vi "OCT with WavePond Clock periodic save updated.vi"() -> ()   [LabVIEW 2014]
doc: "I. Description:\nThis example demonstrates how to acquire a continuous amount of data (Waveform) using the DAQ device's internal clock.\n\nII. Instructions for Running:\n1. Create an analog input voltage channel.\n2. Set the rate for the sample clock. Additionally, define the sample mode to be continuous.\n3. Call the Start VI to start the acquisition.\n4. Read the waveform data in a loop until the user hits the stop button or an error occurs.\nNote: This example reads data from one or more channels and returns an array of data. Use the Index Array function to access an individual channel of data.\n5. Call the Clear Task VI to clear the Task.\n6. Use the popup dialog box to display an error if any.\n\nIV. I/O Connections Overview:\nMake sure your signal input terminal matches the Physical Channel I/O Control. For further connection information, refer to your hardware reference manual."
uses:
  ATS-VI/ATS_ctl/Device_Ctrl.ctl
  ATS-VI/ATS_ctl/ATS_Async_Ctrl.ctl
  ATS-VI/ATS_ctl/ATS_Async_Mode.ctl
  ATS-VI/ATS_ctl/ATS_DMA_Channel.ctl
  ATS-VI/ATS_ctl/ATS_ReadSamples.ctl
  ATS-VI/ATS_ctl/ATS_Check_Ctrl.ctl
  ATS-VI/ATS_ctl/ClockSource.ctl
  Galvo VIs/galvo_states.ctl
  Signal Processing/processing_states.ctl
  En Face/En Face States.ctl
  Saving Data/Saving Data States.ctl
  Type Defs/OCT Hardware States.ctl
  ATS-VI/ATS_ctl/Range.ctl
  ATS-VI/ATS_ctl/Impedance.ctl
  Type Defs/OCT Imaging Parameters Cluster.ctl
  Signal Processing/Display Raw Data states.ctl
  ATS-VI/ATS_ctl/ATS_Spec_Selector.ctl
  Classes/Galvo/Scanning Cluster.ctl
  Classes/Galvo/Galvo.lvclass
  Type Defs/OCT DAQ Channel Data Type.ctl
  Type Defs/Display States.ctl
  ATS-VI/ATS_ctl/Coupling.ctl
  ATS-VI/ATS_ctl/Bandwidth.ctl
  ATS-VI/ATS_ctl/InputCtrl.ctl
  ATS-VI/ATS_ctl/TriggerEngine.ctl
  ATS-VI/ATS_ctl/ExtTrigRange.ctl
  ATS-VI/ATS_ctl/ExtTrigger.ctl
  ATS-VI/ATS_ctl/TriggerOperation.ctl
  ATS-VI/ATS_ctl/Trigger.ctl
  ATS-VI/ATS_ctl/ClockRate.ctl
  ATS-VI/ATS_ctl/ClockEdge.ctl
  ATS-VI/ATS_ctl/Clock.ctl
  ATS-VI/ATS_ctl/Record.ctl
  ATS-VI/ATS_ctl/ATS_Global.ctl
  ATS-VI/ATS_ctl/ATS_Async_Status.ctl
  En Face/En Face Depth Parameters.ctl
  ATS-VI/ATS_ctl/ATS_Async_Setting.ctl
panel:
  in  "update en face image?":bool=TRUE
  in  "total measurement time":dbl=28800.0
  in  "save every ? second":dbl=60.0
  out "First Time?":bool
  out "Save Data":bool
  in  "Async_Setting":T1={"UseHeader"=0, "Rec/Buffer"=200, "Total_Rec"=40000, "DataBuffer"=FALSE, "GetProcessedData"=FALSE}
  out "Processing Finished":bool
  in  "OCT Hardware States":T2=enum."Save Sweep"
  out "Save State":T3=enum."Do Nothing"
  out "Clock Length":u32=9184
  out "Reset DAQ":bool
  in  "Tab Control":T4(tab)=enum."Intensity and Phase B-Scans"
  in  "B-Scans Per Buffer":i32=1
  out "Async_Status":T5={"Start DMA"=TRUE, "StartCapture"=TRUE, "Valid"=TRUE, "Completed"=TRUE, "InProgress"=FALSE, "Timeout"=FALSE, "Overflow"=FALSE, "Error"=FALSE}
  out "Current State":T2
  in  "Channels":tag="Dev1/ao0:1"
  in  "Trigger Source":tag="/Dev1/PFI7"
  in  "Imaging Parameters":T6={"Points Per A-Scan"=1408, "A-Scans per B-Scan"=200, "Voltage Range"=4.0, "Card Resolution (bits)"=16}
  in  "Setup_In":T7={"Record"={"Count"=1, "Presize"=0, "Length"=1408}, "Clock"={"ClckSource"=enum."External", "ClckRate"=17, "ClckEdge"=0, "Decimation"=0}, "Input A"={"Coupling"=enum."DC", "Range"=3, "Impedance"=enum."50 ohms", "Bandwidth"=enum."Full Bandwidth"}, "Input B"={"Coupling"=enum."DC", "Range"=3, "Impedance"=enum."50 ohms", "Bandwidth"=enum."Full Bandwidth"}, "Trigger"={"TrigOperation"=enum."Only X", "Timeout (s)"=1.0, "Trig. Delay"=0, "Engine X"={"Source"=enum."External", "Slope"=enum."Positive", "Level"=150}, "Engine Y"={"Source"=enum."Disable", "Slope"=enum."Positive", "Level"=128}, "ExtTrigControl"={"Coupling"=enum."DC", "Range"=enum."TTL"}}} {"Clock"."ClckEdge" items=["Rising", "Falling"]; "Clock"."ClckRate" items=["1 kS/s", "2 kS/s", "5 kS/s", "10 kS/s", "20 kS/s", "50 kS/s", "100 kS/s", "200 kS/s", "500 kS/s", "1 MS/s", "2 MS/s", "5 MS/s", "10 MS/s", "20 MS/s", "50 MS/s", "100 MS/s", "125 MS/s", "160 MS/s", "180 MS/s"]; "Input B"."Range" items=["200mV", "400mV", "800mV", "2 V", "4 V", "8 V", "16 V"]; "Trigger"."Timeout (s)" format="%.2f"; "Input A"."Range" items=["200mV", "400mV", "800mV", "2 V", "4 V", "8 V", "16 V"]}
  in  "OK Button":bool
  in  "Data Format":T23
  out "Channel A or B Phase (or Channel B Raw)":sgl[][](graph)
  out "Channel A or B Intensity (or Channel A Raw)":sgl[][](graph)
  in  "Display":T24
  out "En Face":dbl[][](graph)
  in  "En Face Parameters":T25={"En Face Start\nDepth"=50, "En Face End\nDepth"=704}
  in  "Save Sweep":bool
  in  "Scanning":T26={"Fast Axis Offset"=200.0, "Slow Axis Offset"=200.0, "Slow Axis Amp"=5.0, "Fast Axis Amp"=5.0, "Scan Pattern"=enum."Raster"} {"Fast Axis Amp" max=20 format="%#.2f"; "Slow Axis Amp" max=20 format="%#.2f"; "Slow Axis Offset" max=10 format="%#.2f"; "Fast Axis Offset" max=10 format="%#.2f"}
  in  "Stop Button":bool
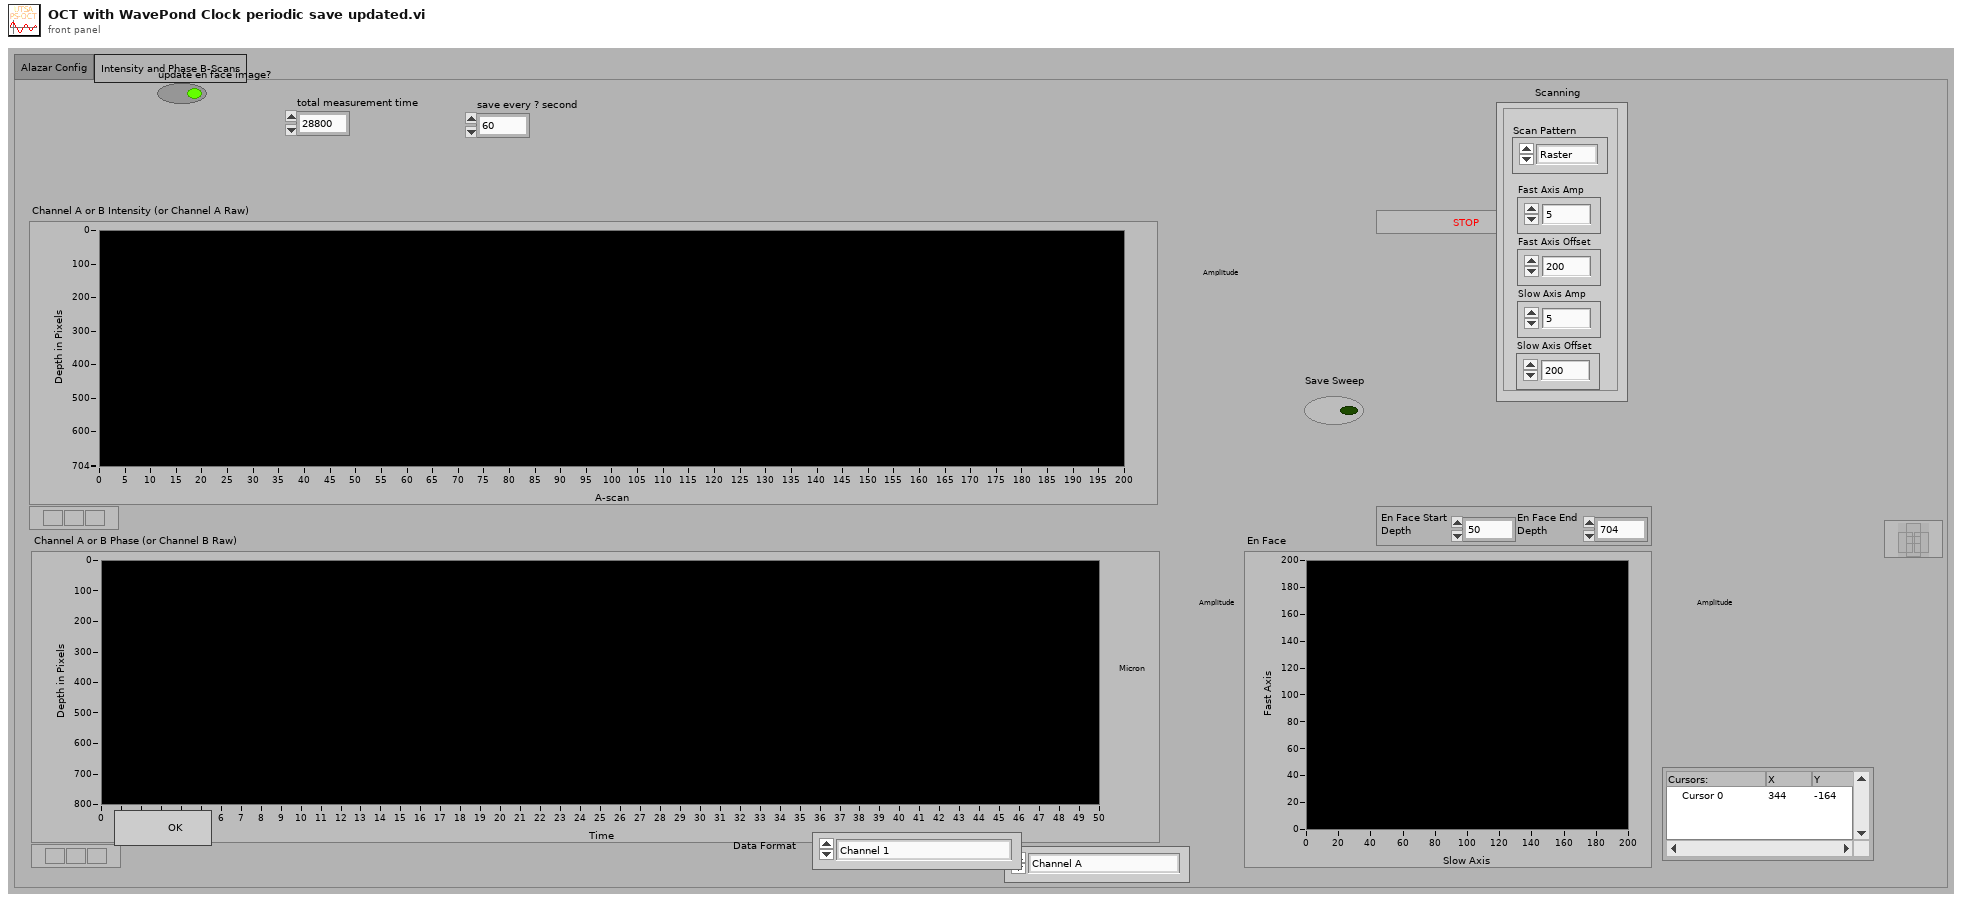
[diagram p1: front panel]
types:
  T1 = typedef "ATS_Async_Setting.ctl" = cluster{"UseHeader":u32, "Rec/Buffer":u32, "Total_Rec":u32, "DataBuffer":bool, "GetProcessedData":bool}
  T2 = typedef "OCT Hardware States.ctl" = enum16{"Acquire Data", "Initialize Laser", "Initialize Galvos", "Startup", "Reset DAQ", "Background Subtraction", "Acquire Background", "Update DAQ Parameters", "Stop", "Set Clock", "Initialize DAQ", "Set Resampling Array", "Save Sweep", "Configure Laser", "128 x 128", "512 x 512", "Review Data"}
  T3 = typedef "Saving Data States.ctl" = enum16{"Get Queue Size", "Get Queue", "Get Timeout", "Flush Queue", "Close Files", "Create Files", "Do Nothing", "Initialize", "Enqueue Data", "Save Data", "Shutdown"}
  T4 = enum32{"Alazar Config", "Intensity and Phase B-Scans"}
  T5 = typedef "ATS_Async_Status.ctl" = cluster{"Start DMA":bool, "StartCapture":bool, "Valid":bool, "Completed":bool, "InProgress":bool, "Timeout":bool, "Overflow":bool, "Error":bool}
  T6 = typedef "OCT Imaging Parameters Cluster.ctl" = cluster{"Points Per A-Scan":i32, "A-Scans per B-Scan":i32, "Voltage Range":sgl, "Card Resolution (bits)":u16}
  T7 = typedef "ATS_Global.ctl" = cluster{"Record":T8, "Clock":T9, "Input A":T13, "Input B":T13, "Trigger":T18}
  T8 = typedef "Record.ctl" = cluster{"Count":u32, "Presize":u32, "Length":u32}
  T9 = typedef "Clock.ctl" = cluster{"ClckSource":T10, "ClckRate":T11, "ClckEdge":T12, "Decimation":u32}
  T10 = typedef "ClockSource.ctl" = enum16{"Internal", "External", "Medium Ext.", "Slow Ext.", "Ext. AC", "Ext. DC", "Ext. (PLL)"}
  T11 = typedef "ClockRate.ctl" = u32
  T12 = typedef "ClockEdge.ctl" = u16
  T13 = typedef "InputCtrl.ctl" = cluster{"Coupling":T14, "Range":T15, "Impedance":T16, "Bandwidth":T17}
  T14 = typedef "Coupling.ctl" = enum16{"AC", "DC"}
  T15 = typedef "Range.ctl" = u32
  T16 = typedef "Impedance.ctl" = enum16{"1M ohms", "50 ohms"}
  T17 = typedef "Bandwidth.ctl" = enum16{"Full Bandwidth", "Reduce Bandwidth"}
  T18 = typedef "Trigger.ctl" = cluster{"TrigOperation":T19, "Timeout (s)":dbl, "Trig. Delay":u32, "Engine X":T20, "Engine Y":T20, "ExtTrigControl":T21}
  T19 = typedef "TriggerOperation.ctl" = enum16{"Only X", "Only Y", "X or Y", "X and Y", "X xor Y", "X and not Y", "not X and Y"}
  T20 = typedef "TriggerEngine.ctl" = cluster{"Source":enum32{"Chan_A", "Chan_B", "External", "Disable"}, "Slope":enum32{"Positive", "Negative"}, "Level":u32}
  T21 = typedef "ExtTrigger.ctl" = cluster{"Coupling":T14, "Range":T22}
  T22 = typedef "ExtTrigRange.ctl" = enum16{"1 V", "5 V", "TTL"}
  T23 = typedef "OCT DAQ Channel Data Type.ctl" = enum16{"Channel 1", "Channel 2", "Channel 1 and 2"}
  T24 = typedef "Display States.ctl" = enum16{"Channel A", "Channel B"}
  T25 = typedef "En Face Depth Parameters.ctl" = cluster{"En Face Start\nDepth":i32, "En Face End\nDepth":i32}
  T26 = typedef "Galvo.lvclass/Scanning Cluster.ctl" = cluster{"Fast Axis Offset":sgl, "Slow Axis Offset":sgl, "Slow Axis Amp":sgl, "Fast Axis Amp":sgl, "Scan Pattern":enum16{"Raster"}}
  T27 = typedef "ATS_Check_Ctrl.ctl" = enum16{"None", "NO_ATS9462", "ATS9462_Traditional", "Verify Board", "OnBoard Memory", "Board & Memory", "Master/Slave", "NO Master/Slave"}
  T28 = typedef "Device_Ctrl.ctl" = enum16{"Status", "About", "Arm", "ForceTrig", "Abort", "Initialize", "Init (NoPreset)", "Info", "Close", "Calibrate", "SetManually", "LED_ON", "LED_OFF"}
  T29 = typedef "ATS_Spec_Selector.ctl" = enum16{"None", "ClckSource", "ClckEdge", "ClckRate", "InputRange", "InputCoupling", "Impedance", "Bandwidth", "AsyncDMA", "Memory", "ExtTrigCoupling", "ExtTrigRange", "AUX_IO_Trig", "AUX_IO_Slope", "Trigger_Source"}
  T30 = typedef "galvo_states.ctl" = enum16{"Reset", "Reset Galvos?", "Center Galvos", "Register Callback", "Get Scan Parameters", "Show", "Initialize", "Run Raster", "Load Raster", "Run Circle", "Shutdown"}
  T31 = typedef "processing_states.ctl" = enum16{"Initialize", "Set Background", "Update Imaging Parameters", "Get Queue", "Process Data", "Get Size", "Flush Data", "Set Reample Array", "Get Last Processed BScan", "Shutdown"}
  T32 = typedef "Display Raw Data states.ctl" = enum16{"Add Raw", "Add Processed", "Show"}
  T33 = typedef "En Face States.ctl" = enum16{"Save BMP", "Show", "Clear En Face", "Update EnFace"}
  T34 = typedef "Processed OCT Data.ctl" = cluster{"Intensity A":sgl[][][], "Phase A":sgl[][][], "Intensity B":sgl[][][], "Phase B":sgl[][][]}
  T35 = enum8{"Enabled", "Disabled", "Disabled and Grayed Out"}
  T36 = typedef "ATS_Async_Ctrl.ctl" = enum16{"SetupDMA", "StartCapture", "Get", "Get_Stream", "Abort", "Stop"}
  T37 = typedef "ATS_ReadSamples.ctl" = cluster{"Offset":i32, "Length":u32}
  T38 = typedef "ATS_DMA_Channel.ctl" = enum16{"Channel_A", "Channel_B", "A & B"}
  T39 = typedef "ATS_Async_Mode.ctl" = enum16{"Continuous", "Triggered", "No-Pre-Trigger", "Traditional"}
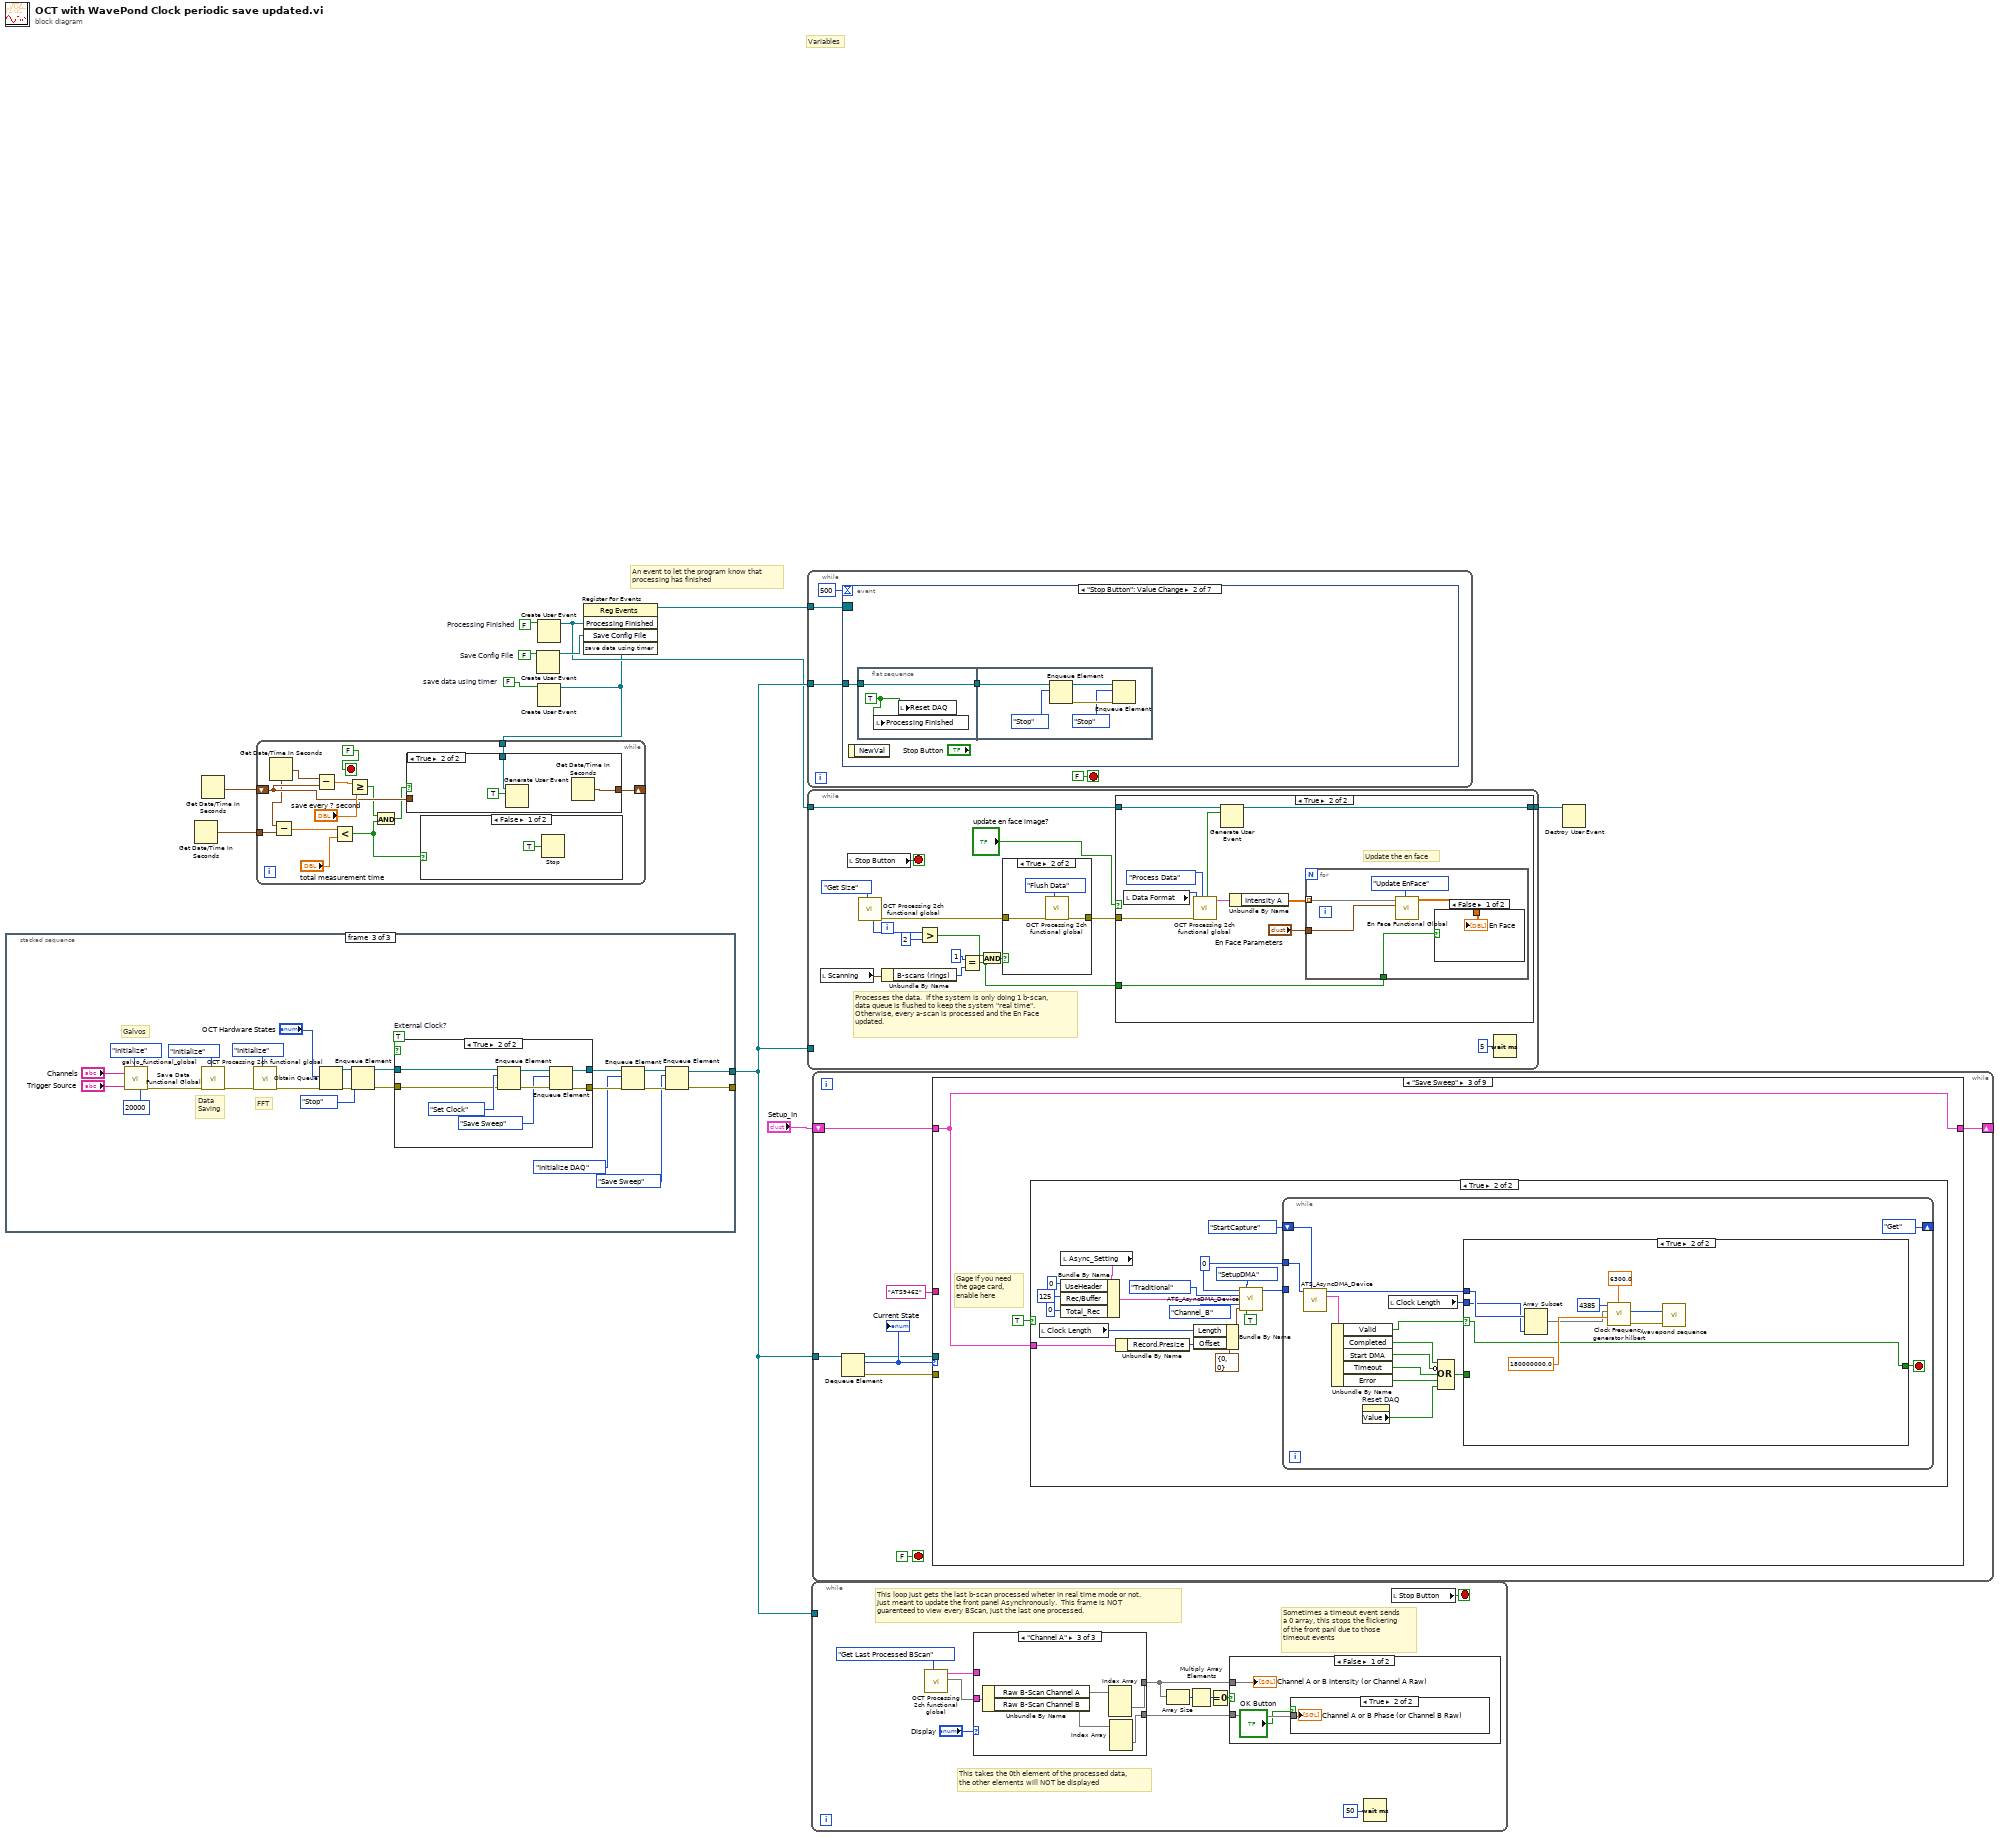
[diagram p0: block diagram]
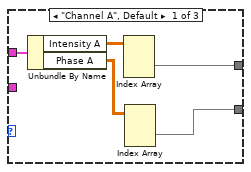
[diagram p9: hidden frame]
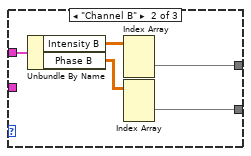
[diagram p10: hidden frame]
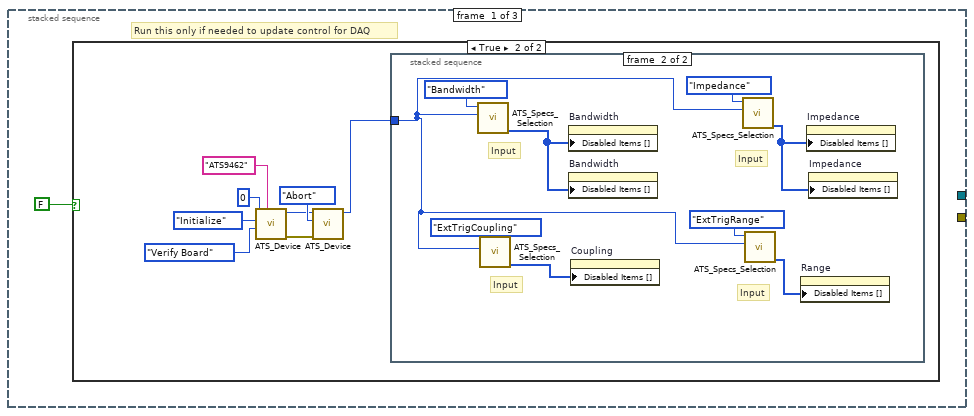
[diagram p11: hidden frame]
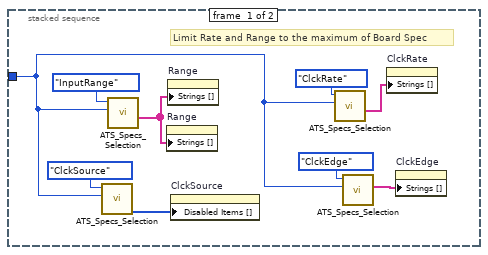
[diagram p13: hidden frame]
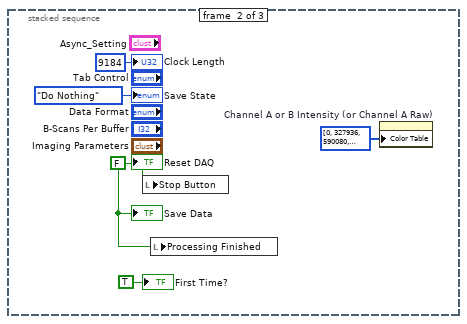
[diagram p14: hidden frame]
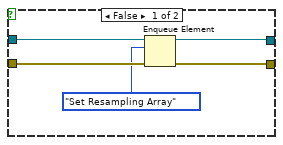
[diagram p15: hidden frame]
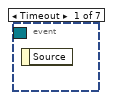
[diagram p16: hidden frame]
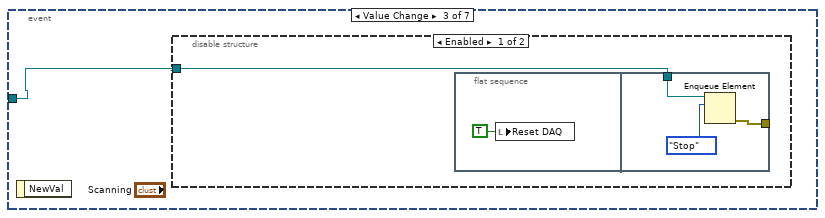
[diagram p17: hidden frame]
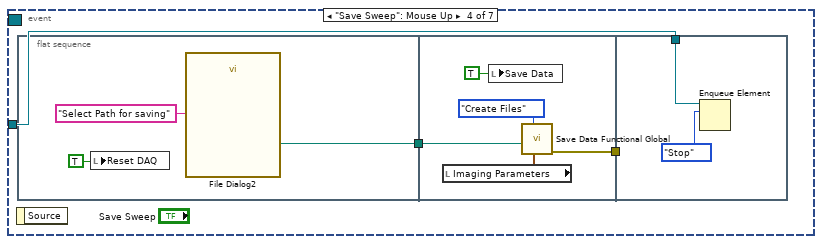
[diagram p19: hidden frame]
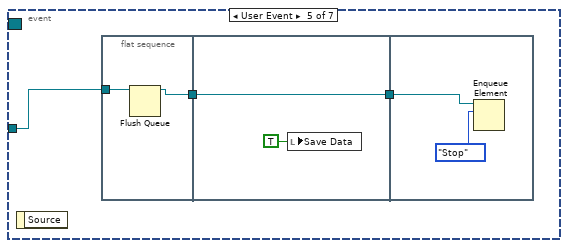
[diagram p20: hidden frame]
diagram:
  w3 = FALSE  # save data using timer
  w4 = FALSE  # Save Config File
  w12 = FALSE  # Processing Finished
  # "An event to let the program know that\nprocessing has finished"
  # "Variables"
  n1 = stacked-sequence {
    tunnel: [_ _ w58] -> _
    tunnel: [_ _ w64] -> w9
    frame #0 {
      # "Run this only if needed to update control for DAQ"
      n2 = case shown="True" FALSE {
        frame False {
        }
        frame True {
          n3 = call "ATS_Device.vi"("BoardToVerify"="ATS9462", "ATS_Check"=ATS_Check_Ctrl."Verify Board", "DevCtrl"=Device_Ctrl."Initialize", "DeviceIn"=0 ("Device")) -> ("error out"=w17:errorcluster, "DeviceOut"=w19:i32)  [unwired: 1 in, 5 out]
          n4 = call "ATS_Device.vi"("error in (no error)"=w17, "DevCtrl"=Device_Ctrl."Abort", "DeviceIn"=w19) -> ("DeviceOut"=w15:i32)  [unwired: 2 in, 6 out]
          n5 = stacked-sequence {
            tunnel: w15 -> [w24 w31]
            frame #0 {
              # "Limit Rate and Range to the maximum of Board Spec"
              n6 = call "ATS_Specs_Selection.vi"("Device"=w24, "ATS_Spec_Selector"=ATS_Spec_Selector."ClckSource") -> ("Disabled_Item"=w23:i32[])  [unwired: 3 in, 6 out]
              n7 = call "ATS_Specs_Selection.vi"("Device"=w24, "ATS_Spec_Selector"=ATS_Spec_Selector."InputRange") -> ("Possible_Item"=w30:string[])  [unwired: 3 in, 6 out]
              n8 = property on="Range" class="Ring (strict)"("Strings []"=w30) -> ()  [unwired: 2 in, 2 out]
              n9 = property on="Range" class="Ring (strict)"("Strings []"=w30) -> ()  [unwired: 2 in, 2 out]
              n10 = property on="ClckSource" class="Enum (strict)"("Disabled Items []"=w23) -> ()  [unwired: 2 in, 2 out]
              n11 = call "ATS_Specs_Selection.vi"("Device"=w24, "ATS_Spec_Selector"=ATS_Spec_Selector."ClckRate") -> ("Possible_Item"=w28:string[])  [unwired: 3 in, 6 out]
              n12 = call "ATS_Specs_Selection.vi"("Device"=w24, "ATS_Spec_Selector"=ATS_Spec_Selector."ClckEdge") -> ("All_Item"=w22:string[])  [unwired: 3 in, 6 out]
              n13 = property on="ClckRate" class="Ring (strict)"("Strings []"=w28) -> ()  [unwired: 2 in, 2 out]
              n14 = property on="ClckEdge" class="Ring (strict)"("Strings []"=w22) -> ()  [unwired: 2 in, 2 out]
            }
            frame #1 {
              # "Input"
              # "Input"
              # "Input"
              # "Input"
              n15 = call "ATS_Specs_Selection.vi"("Device"=w31, "ATS_Spec_Selector"=ATS_Spec_Selector."Bandwidth") -> ("Disabled_Item"=w37:i32[])  [unwired: 3 in, 6 out]
              n16 = call "ATS_Specs_Selection.vi"("Device"=w31, "ATS_Spec_Selector"=ATS_Spec_Selector."ExtTrigCoupling") -> ("Disabled_Item"=w33:i32[])  [unwired: 3 in, 6 out]
              n17 = property on="Bandwidth" class="Enum (strict)"("Disabled Items []"=w37) -> ()  [unwired: 2 in, 2 out]
              n18 = property on="Bandwidth" class="Enum (strict)"("Disabled Items []"=w37) -> ()  [unwired: 2 in, 2 out]
              n19 = property on="Coupling" class="Enum (strict)"("Disabled Items []"=w33) -> ()  [unwired: 2 in, 2 out]
              n20 = call "ATS_Specs_Selection.vi"("Device"=w31, "ATS_Spec_Selector"=ATS_Spec_Selector."Impedance") -> ("Disabled_Item"=w36:i32[])  [unwired: 3 in, 6 out]
              n21 = call "ATS_Specs_Selection.vi"("Device"=w31, "ATS_Spec_Selector"=ATS_Spec_Selector."ExtTrigRange") -> ("Disabled_Item"=w32:i32[])  [unwired: 3 in, 6 out]
              n22 = property on="Range" class="Enum (strict)"("Disabled Items []"=w32) -> ()  [unwired: 2 in, 2 out]
              n23 = property on="Impedance" class="Enum (strict)"("Disabled Items []"=w36) -> ()  [unwired: 2 in, 2 out]
              n24 = property on="Impedance" class="Enum (strict)"("Disabled Items []"=w36) -> ()  [unwired: 2 in, 2 out]
            }
          }
        }
      }
    }
    frame #1 {
      w41 = FALSE ("Sweep Ready for saving")
      n25 = local write "Stop Button"(w41) -> ()
      n26 = local write "Processing Finished"(w41) -> ()
      n27 = property on="Channel A or B Intensity (or Channel A Raw)" class="IntGraph (strict)"("Color Table"=u32[] [0, 327936, 590080, 852224, 983296, 1114624, 1180160, 1311232, 1442304, 1573632, 1704704, 1770240, 1901312, 1966848, 2098176, 2163712, 2294784, 2491392, 2557184, 2688256, 2753792, 2884864, 2950656, 3081728, 3147264, 3344129, 3475457, 3540993, 3672321, 3738113, 3869185, 3934977, 4066305, 4197633, 4328961, 4394497, 4460289, 4591617, 4657409, 4788481, 4854273, 4985601, 5116929, 5248257, 5314049, 5379841, 5511169, 5576961, 5708033, 5773825, 5905153, 6036482, 6167810, 6233346, 6299138, 6430466, 6496258, 6562050, 6693634, 6759426, 6890754, 7022082, 7087874, 7153666, 7284994, 7350786, 7482114, 7547906, 7613698, 7745026, 7876354, 8007682, 8073474, 8139522, 8205314, 8336642, 8467970, 8533763, 8599555, 8665347, 8731139, 8862467, 8993795, 9059587, 9125380, 9191428, 9257220, 9388548, 9454340, 9520132, 9585924, 9717253, 9848837, 9914629, 9980165, 10045957, 10177541, 10243334, 10309126, 10375174, 10440966, 10572294, 10703623, 10769416, 10835208, 10901256, 10967049, 11033097, 11033609, 11099401, 11165450, 11231242, 11231754, 11297547, 11363339, 11429131, 11495180, 11495692, 11561740, 11693069, 11758861, 11759373, 11825165, 11891214, 11957006, 12022799, 12023311, 12089103, 12220944, 12286736, 12286736, 12352529, 12418577, 12484370, 12550162, 12615954, 12681747, 12747796, 12813588, 12813845, 12879894, 12945686, 13077015, 13142808, 13143064, 13208856, 13274905, 13340697, 13340953, 13472282, 13538075, 13604379, 13670172, 13735964, 13801757, 13867550, 13933343, 13999392, 13999648, 14065441, 14131234, 14197027, 14197541, 14263334, 14329383, 14395176, 14460969, 14592553, 14658346, 14724139, 14789932, 14790189, 14856238, 14922287, 14988080, 15053873, 15054130, 15119923, 15185972, 15251765, 15317559, 15383353, 15449146, 15449660, 15515454, 15515968, 15516226, 15582021, 15582278, 15582536, 15648587, 15648844, 15714639, 15714897, 15715155, 15780949, 15781463, 15847256, 15847770, 15848028, 15913823, 15914081, 15979875, 15980133, 15980391, 16046441, 16046444, 16046703, 16046705, 16112500, 16113015, 16113274, 16113277, 16179072, 16179330, 16179588, 16245384, 16245387, 16245389, 16245648, 16311443, 16376982, 16377241, 16377499, 16443294, 16443553, 16443555, 16443815, 16509866, 16510124, 16510127, 16575923, 16575924, 16576182, 16576441, 16576443, 16576702, 16576705, 16576963, 16577222, 16577224, 16577482, 16577485, 16577743, 16577745, 16578004, 16578262, 16578264, 16578523, 16578782, 16579040, 16579299, 16579301, 16579303, 16579562, 16579821]) -> ()  [unwired: 2 in, 2 out]
      "Clock Length" <- u32 9184 ("Clock Length")
      "Save State" <- Saving_Data_States."Do Nothing" ("Save State")
      "Reset DAQ" <- w41
      "Save Data" <- w41
      "First Time?" <- TRUE ("First Time?")
    }
    frame #2 {
      w46 = TRUE  # External Clock?
      # "FFT"
      # "Data \nSaving"
      # "Galvos"
      n28 = call "galvo_functional_global.vi"(4:20000 ("Sweep Speed"), "State"=galvo_states."Initialize", "Trigger Source"="Trigger Source", "Analog Output"="Channels") -> ("error out"=w55:errorcluster)  [unwired: 6 in, 1 out]
      n29 = call "Save Data Functional Global.vi"("States"=Saving_Data_States."Initialize", "error in (no error)"=w55) -> ("error out"=w60:errorcluster)  [unwired: 6 in, 3 out]
      n30 = call "OCT Processing 2ch functional global.vi"("State"=processing_states."Initialize", "error in (no error)"=w60) -> ("error out"=w61:errorcluster)  [unwired: 5 in, 4 out]
      n31 = Obtain Queue(element data type="OCT Hardware States", error in (no error)=w61) -> (queue out=w49:refnum<queue>, error out=w48:errorcluster)  [unwired: 3 in, 1 out]
      n32 = Enqueue Element(queue=w49, element=OCT_Hardware_States."Stop", error in (no error)=w48) -> (queue out=w51:refnum<queue>, error out=w50:errorcluster)  [unwired: 1 in, 1 out]
      n33 = case shown="True" w46 {
        tunnel: [w70 w79] -> w68
        tunnel: [w71 w78] -> w67
        tunnel: w51 -> [w73 w75]
        tunnel: w50 -> [w72 w74]
        frame False {
          n34 = Enqueue Element(queue=w73, element=OCT_Hardware_States."Set Resampling Array", error in (no error)=w72) -> (queue out=w70:refnum<queue>, error out=w71:errorcluster)  [unwired: 1 in, 1 out]
        }
        frame True {
          n35 = Enqueue Element(queue=w75, element=OCT_Hardware_States."Set Clock", error in (no error)=w74) -> (queue out=w81:refnum<queue>, error out=w80:errorcluster)  [unwired: 1 in, 1 out]
          n36 = Enqueue Element(queue=w81, element=OCT_Hardware_States."Save Sweep", error in (no error)=w80) -> (queue out=w79:refnum<queue>, error out=w78:errorcluster)  [unwired: 1 in, 1 out]
        }
      }
      n37 = Enqueue Element(queue=w68, element=OCT_Hardware_States."Initialize DAQ", error in (no error)=w67) -> (queue out=w66:refnum<queue>, error out=w65:errorcluster)  [unwired: 1 in, 1 out]
      n38 = Enqueue Element(queue=w66, element=OCT_Hardware_States."Save Sweep", error in (no error)=w65) -> (queue out=w64:refnum<queue>, error out=w58:errorcluster)  [unwired: 1 in, 1 out]
    }
  }
  n39 = Get Date/Time In Seconds() -> (seconds since 1Jan1904=w1:timestamp)
  n40 = Get Date/Time In Seconds() -> (seconds since 1Jan1904=w5:timestamp)
  n41 = Create User Event(user event datatype=w4) -> (user event=w8:refnum<user-event>)  [unwired: 1 in, 1 out]
  n42 = Create User Event(user event datatype=w12) -> (user event=w7:refnum<user-event>)  [unwired: 1 in, 1 out]
  n43 = Create User Event(user event datatype=w3) -> (user event=w2:refnum<user-event>)  [unwired: 1 in, 1 out]
  n44 = while {
    shift-right: [w91] -> _
    shift-left: w5 -> [w90]
    tunnel: w2 -> [w89]
    tunnel: w1 -> [w87]
    stop <- FALSE stop-if-true
    n45 = Get Date/Time In Seconds() -> (seconds since 1Jan1904=w86:timestamp)
    n46 = Subtract(x=w86, y=w87) -> (x-y=w85:dbl)
    n47 = Subtract(x=w86, y=w90) -> (x-y=w93:dbl)
    n48 = Less?(x=w85, y="total measurement time") -> (x < y?=w82:bool)
    n49 = Greater Or Equal?(x=w93, y="save every ? second") -> (x >= y?=w84:bool)
    n50 = And(x=w84, y=w82) -> (x .and. y?=w83:bool)
    n51 = case shown="True" w83 {
      tunnel: [w96 w99] -> w91
      tunnel: w90 -> [w96 _]
      tunnel: w89 -> [_ w98]
      frame False {
      }
      frame True {
        n52 = Generate User Event(user event=w98, event data cluster=TRUE ("event data")) -> ()  [unwired: 2 in, 2 out]
        n53 = Get Date/Time In Seconds() -> (seconds since 1Jan1904=w99:timestamp)
      }
    }
    n54 = case shown="False" w82 {
      frame False {
        n55 = Stop(stop? (T)=TRUE) -> ()
      }
      frame True {
      }
    }
  }
  n56 = register-events(w7, w8, w2) -> (reference out=w11:refnum<event-registration>)  [unwired: 2 in, 1 out]
  n57 = while {
    tunnel: w9 -> [w101]
    tunnel: w11 -> [w102]
    stop <- FALSE stop-if-true
    n58 = event shown="[1] \"Stop Button\": Value Change" {
      selector: w102 -> [_ _ _ _ _ _ _]
      dyn-events: _ -> [_ _ _ _ _ _ _]
      timeout: 500 -> [_ _ _ _ _ _ _]
      tunnel: w101 -> [_ w104 w113 w121 w132 _ _]
      event Timeout {
        n59 = event-data() -> ()  [unwired: 1 in, 1 out]
      }
      event "Stop Button": Value Change {
        n60 = event-data() -> ()  [unwired: 1 in, 1 out]
        n61 = flat-sequence {
          tunnel: w104 -> [w107]
          tunnel: [w107] -> w105
          tunnel: w105 -> [w112]
          frame #0 {
            w106 = TRUE ("Reset DAQ")
            n62 = local write "Processing Finished"(w106) -> ()
            n63 = local write "Reset DAQ"(w106) -> ()
          }
          frame #1 {
            n64 = Enqueue Element(queue=w112, element=OCT_Hardware_States."Stop") -> (queue out=w109:refnum<queue>, error out=w110:errorcluster)  [unwired: 2 in, 1 out]
            n65 = Enqueue Element(queue=w109, element=OCT_Hardware_States."Stop", error in (no error)=w110) -> ()  [unwired: 1 in, 3 out]
          }
        }
      }
      event Value Change {
        n66 = event-data() -> ()  [unwired: 1 in, 1 out]
        n67 = disable-structure shown="Enabled" {
          disable-tunnel: w113 -> [w114 _]
          frame Enabled {
            n68 = flat-sequence {
              tunnel: w114 -> [w117]
              tunnel: [w116] -> _
              frame #0 {
                n69 = local write "Reset DAQ"(TRUE ("Reset DAQ")) -> ()
              }
              frame #1 {
                n70 = Enqueue Element(queue=w117, element=OCT_Hardware_States."Stop") -> (error out=w116:errorcluster)  [unwired: 2 in, 2 out]
              }
            }
          }
          frame Disabled {
          }
        }
      }
      event "Save Sweep": Mouse Up {
        n71 = event-data() -> ()  [unwired: 1 in, 1 out]
        n72 = flat-sequence {
          tunnel: [w122] -> w120
          tunnel: w120 -> [w129]
          tunnel: [w127] -> w119
          tunnel: w121 -> [w131]
          tunnel: w119 -> [_]
          frame #0 {
            n73 = local write "Reset DAQ"(TRUE ("Reset DAQ")) -> ()
            n74 = call "File Dialog2"("prompt"="Select Path for saving") -> ("selected path"=w122:path)  [unwired: 11 in, 3 out]
          }
          frame #1 {
            n75 = local read "Imaging Parameters"() -> (w126:T6)
            n76 = local write "Save Data"(TRUE ("Save Data")) -> ()
            n77 = call "Save Data Functional Global.vi"("Input Parameters"=w126, "States"=Saving_Data_States."Create Files", "Folder"=w129) -> ("error out"=w127:errorcluster)  [unwired: 5 in, 3 out]
          }
          frame #2 {
            n78 = Enqueue Element(queue=w131, element=OCT_Hardware_States."Stop") -> ()  [unwired: 2 in, 3 out]
          }
        }
      }
      event User Event {
        n79 = event-data() -> ()  [unwired: 1 in, 1 out]
        n80 = flat-sequence {
          tunnel: [w136] -> w133
          tunnel: w132 -> [w135]
          tunnel: [w138] -> w134
          tunnel: w133 -> [w138]
          tunnel: w134 -> [w139]
          frame #0 {
            n81 = Flush Queue(queue=w135) -> (queue out=w136:refnum<queue>)  [unwired: 1 in, 2 out]
          }
          frame #1 {
            n82 = local write "Save Data"(TRUE ("Save Data")) -> ()
          }
          frame #2 {
            n83 = Enqueue Element(queue=w139, element=OCT_Hardware_States."Stop") -> ()  [unwired: 2 in, 3 out]
          }
        }
      }
      event User Event {
        n84 = event-data() -> ()  [unwired: 1 in, 1 out]
        n85 = call "OCT Processing 2ch functional global.vi"("State"=processing_states."Get Size") -> ("# elements in queue"=w142:i32)  [unwired: 6 in, 4 out]
        n86 = Equal To 0?(x=w142) -> (x = 0?=→"Processing Finished":bool)
      }
      event Menu Selection (User) {
        n87 = event-data() -> ("ItemTag"=w144:string)  [unwired: 1 in, 2 out]
        n88 = case shown="\"Raw Data\", Default" w144 {
          frame "Raw Data", Default {
            n89 = call "Display Raw Data.vi"("Enum"=Display_Raw_Data_states."Show") -> ()  [unwired: 11 in]
          }
        }
      }
    }
  }
  n90 = while {
    tunnel: w7 -> [w152]
    tunnel: [w151] -> w10
    tunnel: w9 -> [_]
    stop <- w161 stop-if-true
    # "Processes the data.  If the system is only doing 1 b-scan, \ndata queue is flushed to keep the system \"real time\".\nOtherwise, every a-scan is processed and the En Face\nupdated."
    n91 = local read "Scanning"() -> (w154:T26)
    n92 = local read "Stop Button"() -> (w161:bool)
    n93 = call "OCT Processing 2ch functional global.vi"("State"=processing_states."Get Size") -> ("error out"=w150:errorcluster, "# elements in queue"=w158:i32)  [unwired: 6 in, 3 out]
    n94 = Unbundle By Name(w154) -> ("B-scans (rings)"=w153:u32)
    n95 = Greater?(x=w158, y=2) -> (0:w159:bool)
    n96 = Equal?(x=u32 1, y=w153) -> (x = y?=w147:bool)
    n97 = And(x=w159, y=w147) -> (x .and. y?=w148:bool)
    n98 = case shown="True" w148 {
      tunnel: w150 -> [w179 w182]
      tunnel: [w179 w181] -> w149
      frame False {
      }
      frame True {
        n99 = call "OCT Processing 2ch functional global.vi"("State"=processing_states."Flush Data", "error in (no error)"=w182) -> ("error out"=w181:errorcluster)  [unwired: 5 in, 4 out]
      }
    }
    n100 = case shown="True" "update en face image?" {
      tunnel: w152 -> [w162 w169]
      tunnel: [w162 w167] -> w151
      tunnel: w149 -> [_ w164]
      tunnel: w147 -> [_ w163]
      frame False {
      }
      frame True {
        # "Update the en face"
        n101 = local read "Data Format"() -> (w170:T23)
        n102 = call "OCT Processing 2ch functional global.vi"("State"=processing_states."Process Data", "error in (no error)"=w164, "Data Format"=w170) -> ("Processed OCT Data"=w171:T34, "Time Out"=w168:bool)  [unwired: 4 in, 3 out]
        n103 = Generate User Event(user event=w169, event data cluster=w168) -> (user event out=w167:refnum<user-event>)  [unwired: 2 in, 1 out]
        n104 = Unbundle By Name(w171) -> ("Intensity A"=w165:sgl[][][])
        n105 = for {
          tunnel: "En Face Parameters" -> [w176]
          tunnel: w165 -> [w175] mode=indexing
          tunnel: w163 -> [w173]
          n106 = call "En Face Functional Global.vi"(7:En_Face_States."Update EnFace" ("En Face States"), 10:w176, "Intensity Graph 2"=w175) -> ("Intensity Graph"=w174:dbl[][])  [unwired: 7 in, 1 out]
          n107 = case shown="False" w173 {
            tunnel: w174 -> [w178 _]
            frame False {
              "En Face" <- w178
            }
            frame True {
            }
          }
        }
      }
    }
    n108 = Wait (ms)(milliseconds to wait=u32 5) -> ()  [unwired: 1 out]
  }
  n109 = while {
    tunnel: w9 -> [_]
    stop <- w193 stop-if-true
    # "Sometimes a timeout event sends\na 0 array, this stops the flickering\nof the front panl due to those \ntimeout events"
    # "This takes the 0th element of the processed data,\nthe other elements will NOT be displayed"
    # "This loop just gets the last b-scan processed wheter in real time mode or not. \nJust meant to update the front panel Asynchronously.  This frame is NOT\nguarenteed to view every BScan, just the last one processed."
    n110 = call "OCT Processing 2ch functional global.vi"("State"=processing_states."Get Last Processed BScan") -> (2:w189, "Processed OCT Data"=w187:T34)  [unwired: 5 in, 4 out]
    n111 = case shown="\"Raw Data A and B\"" "Display" {
      tunnel: w187 -> [w202 w203 _]
      tunnel: w189 -> [_ _ w212]
      tunnel: [w198 w205 w210] -> w185
      tunnel: [w199 w204 w209] -> w188
      frame "Channel A", Default {
        n112 = Unbundle By Name(w202) -> ("Intensity A"=w200:sgl[][][], "Phase A"=w201:sgl[][][])
        n113 = Index Array(array=w200) -> (element=w198:sgl[][])  [unwired: 3 in]
        n114 = Index Array(array=w201) -> (element=w199:sgl[][])  [unwired: 3 in]
      }
      frame "Channel B" {
        n115 = Unbundle By Name(w203) -> ("Intensity B"=w206:sgl[][][], "Phase B"=w207:sgl[][][])
        n116 = Index Array(array=w206) -> (element=w205:sgl[][])  [unwired: 3 in]
        n117 = Index Array(array=w207) -> (element=w204:sgl[][])  [unwired: 3 in]
      }
      frame "Channel A" {
        n118 = Unbundle By Name(w212) -> ("Raw B-Scan Channel A"=w208, "Raw B-Scan Channel B"=w211)
        n119 = Index Array(array=w208) -> (element=w210)  [unwired: 3 in]
        n120 = Index Array(array=w211) -> (element=w209)  [unwired: 3 in]
      }
    }
    n121 = Array Size(array=w185) -> (size(s)=w186:i32[])
    n122 = Multiply Array Elements(1:w186) -> (0:w184:i32)
    n123 = Equal To 0?(x=w184) -> (x = 0?=w183:bool)
    n124 = case shown="False" w183 {
      tunnel: w188 -> [w196 _]
      tunnel: w185 -> [w195 _]
      frame False {
        n125 = case shown="True" "OK Button" {
          tunnel: w196 -> [_ w197]
          frame False {
          }
          frame True {
            "Channel A or B Phase (or Channel B Raw)" <- w197
          }
        }
        "Channel A or B Intensity (or Channel A Raw)" <- w195
      }
      frame True {
      }
    }
    n126 = Wait (ms)(milliseconds to wait=u32 50) -> ()  [unwired: 1 out]
    n127 = local read "Stop Button"() -> (w193:bool)
  }
  n128 = while {
    tunnel: w9 -> [w220]
    shift-right: [w214] -> _
    shift-left: "Setup_In" -> [w213]
    stop <- FALSE stop-if-true
    n129 = Dequeue Element(queue=w220) -> (queue out=w216:refnum<queue>, element=w218:T2, error out=w217:errorcluster)  [unwired: 2 in, 1 out]
    "Current State" <- w218
    n130 = case shown="\"Save Sweep\"" w218 {
      tunnel: w217 -> [w234 w250 _ _ w351 w402 _ w483 _]
      tunnel: w216 -> [w233 w252 _ _ w360 w425 _ w484 _]
      tunnel: "ATS9462" ("BoardToVerify") -> [_ _ _ w312 _ _ _ _ w491]
      tunnel: [w232 w247 w262 w306 w347 w407 w473 w475 w490] -> w214
      tunnel: w213 -> [w232 w247 w262 w305 w347 w407 w473 w475 w490]
      frame "Save Sweep" {
        n131 = call "galvo_functional_global.vi"("State"=galvo_states."Reset", "error in (no error)"=w234) -> ("error out"=w222:errorcluster)  [unwired: 8 in, 1 out]
        n132 = local read "Scanning"() -> (w224:T26)
        n133 = local read "B-Scans Per Buffer"() -> (w225:i32)
        n134 = call "galvo_functional_global.vi"("Est Sweep Speed"=w225, "State"=galvo_states."Load Raster", "error in (no error)"=w222, "user event out"=w224) -> ("error out"=w221:errorcluster)  [unwired: 6 in, 1 out]
        n135 = Enqueue Element(queue=w233, element=OCT_Hardware_States."Initialize DAQ", error in (no error)=w221) -> (queue out=w230:refnum<queue>, error out=w229:errorcluster)  [unwired: 1 in, 1 out]
        n136 = local read "Save Data"() -> (w228:bool)
        n137 = case shown="True" w228 {
          tunnel: w230 -> [w237 w242]
          tunnel: w229 -> [w236 w241]
          tunnel: [FALSE ("Reset DAQ") FALSE ("Reset DAQ")] -> w227
          frame False {
            n138 = Enqueue Element(queue=w237, element=OCT_Hardware_States."Acquire Data", error in (no error)=w236) -> ()  [unwired: 1 in, 3 out]
          }
          frame True {
            n139 = Enqueue Element(queue=w242, element=OCT_Hardware_States."Acquire Data", error in (no error)=w241) -> ()  [unwired: 1 in, 3 out]
          }
        }
        n140 = local write "Save Data"(w227) -> ()
      }
      frame "Stop" {
        n141 = flat-sequence {
          tunnel: w250 -> [w260]
          tunnel: [w260] -> w249
          frame #0 {
            n142 = local write "Processing Finished"(FALSE ("Reset DAQ")) -> ()
            n143 = local write "Reset DAQ"(FALSE ("Reset DAQ")) -> ()
          }
        }
        n144 = call "Save Data Functional Global.vi"("States"=Saving_Data_States."Flush Queue", "error in (no error)"=w249) -> ("error out"=w243:errorcluster)  [unwired: 6 in, 3 out]
        n145 = call "OCT Processing 2ch functional global.vi"("State"=processing_states."Flush Data", "error in (no error)"=w243) -> ("error out"=w246:errorcluster)  [unwired: 5 in, 4 out]
        n146 = property on="Save Sweep" class="Bool"(error in=w246, "DisabledEnum"=T35."Disabled and Grayed Out" ("Disabled")) -> (error out=w245:errorcluster)  [unwired: 1 in, 1 out]
        n147 = Enqueue Element(queue=w252, element=OCT_Hardware_States."Save Sweep", error in (no error)=w245) -> (error out=w248:errorcluster)  [unwired: 1 in, 2 out]
        n148 = flat-sequence {
          tunnel: w248 -> [_]
          frame #0 {
            w258 = 0 ("DeviceIn")
            n149 = call "ATS_AsyncDMA_Device.vi"("DeviceIn"=w258, "ATS_Async_Ctrl"=ATS_Async_Ctrl."Stop") -> ("ReadSamples_Out"=w257:T37)  [unwired: 9 in, 4 out]
            n150 = call "ATS_AsyncDMA_Device.vi"("DeviceIn"=w258, "ATS_Async_Ctrl"=ATS_Async_Ctrl."Abort", "ReadSamples"=w257) -> ()  [unwired: 8 in, 5 out]
          }
        }
      }
      frame "Save Sweep" {
        # "Gage if you need\nthe gage card,\nenable here"
        n151 = case shown="True" TRUE {
          tunnel: w262 -> [_ w264]
          frame False {
          }
          frame True {
            w268 = 0 ("DeviceIn")
            n152 = local read "Clock Length"() -> (w270:u32)
            n153 = local read "Async_Setting"() -> (w266:T1)
            n154 = Bundle By Name(cluster=w266, "UseHeader"=u32 0, "Rec/Buffer"=u32 125, "Total_Rec"=u32 0) -> (w267:T1)
            n155 = Unbundle By Name(w264) -> ("Record.Presize"=w271:u32)
            n156 = Bundle By Name(cluster=T37 {"Offset"=0, "Length"=0} ("ReadSamples"), "Length"=w270, "Offset"=w271) -> (w269:T37)
            n157 = call "ATS_AsyncDMA_Device.vi"("DeviceIn"=w268, "ATS_Async_Ctrl"=ATS_Async_Ctrl."SetupDMA" ("ATS_DMA_Ctrl"), "Async_Mode"=ATS_Async_Mode."Traditional", "Async_Setting"=w267, "Channel"=ATS_DMA_Channel."Channel_B", "ReadSamples"=w269, "Start Now / Wait"=TRUE) -> ("Buffer"=w276:u16[])  [unwired: 4 in, 4 out]
            n158 = while {
              tunnel: w276 -> [_]
              shift-right: [ATS_Async_Ctrl."Get" ("ATS_Async_Ctrl")] -> _
              shift-left: ATS_Async_Ctrl."StartCapture" ("ATS_Async_Ctrl") -> [w290]
              tunnel: w268 -> [w284]
              stop <- w287 stop-if-true
              n159 = call "ATS_AsyncDMA_Device.vi"("DeviceIn"=w284, "ATS_Async_Ctrl"=w290) -> ("Buffer"=w282:u16[], "Async_Status"=w281:T5)  [unwired: 9 in, 3 out]
              n160 = Unbundle By Name(w281) -> ("Valid"=w283:bool, "Completed"=w292:bool, "Start DMA"=w293:bool, "Timeout"=w294:bool, "Error"=w291:bool)
              n161 = property on="Reset DAQ" class="Bool (strict)"() -> ("Value"=w288:bool)  [unwired: 2 in, 2 out]
              n162 = local read "Clock Length"() -> (w285:u32)
              n163 = Compound Arithmetic op=OR(w292, invert w293, w294, w291, w288) -> (w286:bool)
              n164 = case shown="True" w283 {
                selector: w283 -> [w295 w298]
                tunnel: w282 -> [_ w297]
                tunnel: [w295 w298] -> w287
                tunnel: w286 -> [_ _]
                tunnel: w285 -> [_ w296]
                frame False {
                }
                frame True {
                  n165 = Array Subset(array=w297, length=w296) -> (w299:u16[])  [unwired: 1 in]
                  n166 = call "Clock Frequency generator hilbert.vi"(7:6300.0 ("Sweep Speed"), "Acquisition speed (S/s)"=180000000.0 ("Sweep Speed"), "k-space signal in"=w299, "number of frequency updates"=4385) -> ("Error Out"=w304:errorcluster, "frequency\nsteps"=w303:i32)  [unwired: 6 in]
                  n167 = call "wavepond sequence.vi"("Error In"=w304, "Number of updates"=w303) -> ()  [unwired: 9 in, 1 out]
                }
              }
            }
          }
        }
      }
      frame "Initialize DAQ" {
        # "B-Scans per buffer should be around 4 if \ntaking more than 1 to minimize data transfer"
        # "If B Scans is 1, set total records to 0,\notherwise it should be A-Scans Per\nBScan times BScans"
        # "BScans Per Buffer"
        n168 = local read "First Time?"() -> (w309:bool)
        n169 = case shown="True" w309 {
          tunnel: [_ w341] -> w335
          tunnel: w312 -> [_ w337]
          tunnel: [FALSE ("First Time?") FALSE ("First Time?")] -> w308
          frame False {
          }
          frame True {
            n170 = call "ATS_Device.vi"("BoardToVerify"=w337, "ATS_Check"=ATS_Check_Ctrl."Verify Board", "DevCtrl"=Device_Ctrl."Initialize", "DeviceIn"=0 ("Device")) -> ("error out"=w339:errorcluster, "DeviceOut"=w343:i32)  [unwired: 1 in, 5 out]
            n171 = call "ATS_Device.vi"("error in (no error)"=w339, "DevCtrl"=Device_Ctrl."Abort", "DeviceIn"=w343) -> ("DeviceOut"=w341:i32)  [unwired: 2 in, 6 out]
          }
        }
        n172 = local write "First Time?"(w308) -> ()
        n173 = Unbundle By Name(w305) -> ("Record.Length"=w313:u32)
        n174 = call "ATS_MS_Set_Device.vi"("Set_Manually (F)"=FALSE, "Setup_In"=w305, "DeviceIn"=w335) -> ("Setup_Out"=w306:T7)  [unwired: 3 in, 5 out]
        n175 = local read "Scanning"() -> (w331:T26)
        n176 = Unbundle By Name(w331) -> ("B-scans (rings)"=w319:u32, "A(cluster)/B"=w329:u32, "B-scans (rings)"=w324:u32, "A(cluster)/B"=w323:u32, "B-scans (rings)"=w321:u32, "A(cluster)/B"=w315:u32)
        n177 = Not Equal?(x=w321, y=u32 1 ("x")) -> (x != y?=w322:bool)
        n178 = Equal?(x=u32 1, y=w319) -> (x = y?=w325:bool)
        n179 = local read "B-Scans Per Buffer"() -> (w307:i32)
        n180 = Select(t=u32 4 ("y"), s=w325, f=w307) -> (s? t:f=w327:u32)
        n181 = Multiply(x=w324, y=w323) -> (x*y=w318:u32)
        n182 = local read "Async_Setting"() -> (w311:T1)
        n183 = Select(t=w318, s=w322, f=u32 0 ("Total_Rec")) -> (s? t:f=w333:u32)
        n184 = Multiply(x=w327, y=w329) -> (x*y=w330:u32)
        n185 = Bundle By Name(cluster=T6 {"Points Per A-Scan"=0, "A-Scans per B-Scan"=0, "Voltage Range"=4.0, "Card Resolution (bits)"=16} ("Imaging Parameters"), "Points Per A-Scan"=w313, "A-Scans per B-Scan"=w315) -> (w314:T6)
        n186 = Bundle By Name(cluster=w311, "UseHeader"=u32 0, "Rec/Buffer"=w330, "Total_Rec"=w333) -> (w310:T1)
        n187 = local write "Async_Setting"(w310) -> ()
        n188 = local write "Imaging Parameters"(w314) -> ()
      }
      frame "Acquire Data", Default {
        w368 = 0 ("DeviceIn")
        # "Update and \nclear the \nEn Face"
        # "Tell the FFT the most\nup-to-date imaging\nparameters"
        n189 = Enqueue Element(queue=w360, element=OCT_Hardware_States."Stop", error in (no error)=w351) -> (error out=w350:errorcluster)  [unwired: 1 in, 2 out]
        n190 = local read "Imaging Parameters"() -> (w357:T6)
        n191 = local read "Data Format"() -> (w362:T23)
        n192 = local read "Async_Setting"() -> (w355:T1)
        n193 = case shown="\"Channel 1\", Default" w362 {
          tunnel: [ATS_DMA_Channel."Channel_A" ("Channel") ATS_DMA_Channel."A & B" ("Channel") ATS_DMA_Channel."A & B" ("Channel")] -> w361
          frame "Channel 1", Default {
          }
          frame "Channel 2" {
          }
          frame "Channel 1 and 2" {
          }
        }
        n194 = call "OCT Processing 2ch functional global.vi"("State"=processing_states."Update Imaging Parameters", "error in (no error)"=w350, "Input Parameters"=w357) -> ("error out"=w359:errorcluster)  [unwired: 4 in, 4 out]
        n195 = local read "Scanning"() -> (w354:T26)
        n196 = call "En Face Functional Global.vi"(7:En_Face_States."Clear En Face" ("En Face States"), "Error In"=w359, 9:w354) -> ("Error Out"=w353:errorcluster)  [unwired: 7 in, 1 out]
        n197 = Unbundle By Name(w347) -> ("Record.Length"=w364:u32, "Record.Presize"=w363:u32)
        n198 = Unbundle By Name(w347) -> ("Record.Length"=w346:u32)
        n199 = call "OCT Processing 2ch functional global.vi"("State"=processing_states."Get Queue", "error in (no error)"=w353) -> ("queue out"=w349:refnum<queue>)  [unwired: 5 in, 4 out]
        n200 = Bundle By Name(cluster=T37 {"Offset"=0, "Length"=0} ("ReadSamples"), "Length"=w364, "Offset"=w363) -> (w370:T37)
        n201 = call "ATS_AsyncDMA_Device.vi"("DeviceIn"=w368, "ATS_Async_Ctrl"=ATS_Async_Ctrl."SetupDMA" ("ATS_DMA_Ctrl"), "Async_Mode"=ATS_Async_Mode."No-Pre-Trigger", "Async_Setting"=w355, "Channel"=w361, "ReadSamples"=w370, "Start Now / Wait"=TRUE) -> ("Buffer"=w366:u16[])  [unwired: 4 in, 4 out]
        n202 = while {
          tunnel: w366 -> [_]
          tunnel: w368 -> [w394]
          shift-right: [ATS_Async_Ctrl."Get" ("ATS_Async_Ctrl")] -> _
          shift-left: ATS_Async_Ctrl."StartCapture" ("ATS_Async_Ctrl") -> [w391]
          tunnel: w349 -> [w383]
          tunnel: [w382] -> w348
          tunnel: w346 -> [w381]
          stop <- w382 stop-if-true
          n203 = call "ATS_AsyncDMA_Device.vi"("DeviceIn"=w394, "ATS_Async_Ctrl"=w391) -> ("Buffer"=w387:u16[], "Async_Status"=w389:T5)  [unwired: 9 in, 3 out]
          "Async_Status" <- w389
          n204 = Unbundle By Name(w389) -> ("Valid"=w388:bool, "Completed"=w384:bool, "Start DMA"=w385:bool, "Timeout"=w393:bool, "Error"=w392:bool)
          n205 = local read "Reset DAQ"() -> (w386:bool)
          n206 = Compound Arithmetic op=OR(w384, invert w385, w393, w392, w386) -> (w382:bool)
          n207 = case shown="True" w388 {
            tunnel: w387 -> [_ w399]
            tunnel: w383 -> [_ w401]
            tunnel: w381 -> [_ w398]
            frame False {
              # "Do nothing"
            }
            frame True {
              n208 = Enqueue Element(queue=w401, element=w399, timeout in ms (-1)=50) -> (error out=w396:errorcluster)  [unwired: 1 in, 2 out]
              n209 = property on="Save Sweep" class="Bool"(error in=w396, "DisabledEnum"=T35."Enabled" ("Disabled")) -> ()  [unwired: 1 in, 2 out]
              n210 = call "Display Raw Data.vi"("Enum"=Display_Raw_Data_states."Add Processed", "Length"=w398, "Raw Data In"=w399) -> ()  [unwired: 9 in]
            }
          }
        }
        n211 = while {
          tunnel: w348 -> [w377]
          stop <- w375 stop-if-true
          n212 = local read "Processing Finished"() -> (w376:bool)
          n213 = Wait (ms)(milliseconds to wait=u32 50) -> ()  [unwired: 1 out]
          n214 = And(x=w377, y=w376) -> (x .and. y?=w375:bool)
        }
      }
      frame "Acquire Data" {
        w433 = 0 ("DeviceIn")
        # "Close files and set save \nstate to do nothing"
        # "Update and \nclear the \nEn Face"
        # "Tell the FFT the most\nup-to-date imaging\nparameters"
        n215 = local read "Imaging Parameters"() -> (w422:T6)
        n216 = local read "Imaging Parameters"() -> (w405:T6)
        n217 = local read "Data Format"() -> (w427:T23)
        n218 = local read "Async_Setting"() -> (w416:T1)
        n219 = case shown="\"Channel 1\", Default" w427 {
          tunnel: [ATS_DMA_Channel."Channel_A" ("Channel") ATS_DMA_Channel."A & B" ("Channel") ATS_DMA_Channel."A & B" ("Channel")] -> w426
          frame "Channel 1", Default {
          }
          frame "Channel 2" {
          }
          frame "Channel 1 and 2" {
          }
        }
        n220 = call "Save Data Functional Global.vi"("Input Parameters"=w405, "States"=Saving_Data_States."Create Files", "error in (no error)"=w402, "Folder"=path "D:/Worm" ("selected path")) -> ("error out"=w403:errorcluster)  [unwired: 4 in, 3 out]
        n221 = call "OCT Processing 2ch functional global.vi"("State"=processing_states."Update Imaging Parameters", "error in (no error)"=w402, "Input Parameters"=w422) -> ("error out"=w424:errorcluster)  [unwired: 4 in, 4 out]
        n222 = local read "Scanning"() -> (w415:T26)
        n223 = call "En Face Functional Global.vi"(7:En_Face_States."Clear En Face" ("En Face States"), "Error In"=w424, 9:w415) -> ("Error Out"=w414:errorcluster)  [unwired: 7 in, 1 out]
        n224 = Unbundle By Name(w407) -> ("Record.Length"=w429:u32, "Record.Presize"=w428:u32)
        n225 = call "Save Data Functional Global.vi"("States"=Saving_Data_States."Get Queue", "error in (no error)"=w403) -> ("Saving Queue Out"=w409:refnum<queue>)  [unwired: 6 in, 3 out]
        n226 = call "OCT Processing 2ch functional global.vi"("State"=processing_states."Get Queue", "error in (no error)"=w414) -> ("error out"=w413:errorcluster, "queue out"=w411:refnum<queue>)  [unwired: 5 in, 3 out]
        n227 = Bundle By Name(cluster=T37 {"Offset"=0, "Length"=0} ("ReadSamples"), "Length"=w429, "Offset"=w428) -> (w435:T37)
        n228 = call "ATS_AsyncDMA_Device.vi"("DeviceIn"=w433, "ATS_Async_Ctrl"=ATS_Async_Ctrl."SetupDMA" ("ATS_DMA_Ctrl"), "Async_Mode"=ATS_Async_Mode."No-Pre-Trigger", "Async_Setting"=w416, "Channel"=w426, "ReadSamples"=w435, "Start Now / Wait"=TRUE) -> ("Buffer"=w431:u16[])  [unwired: 4 in, 4 out]
        n229 = while {
          tunnel: w413 -> [_]
          tunnel: [w444] -> w421
          i -> [w443]
          stop <- w442 stop-if-true
          # "Saves data as long as data is being fed into the Queue,\notherwise it will time out and halt this loop."
          n230 = case shown="1, Default" w443 {
            tunnel: [FALSE w450] -> w442
            tunnel: [_ w447] -> w444
            frame 0 {
              # "Wait for data to Q up"
              n231 = Wait (ms)(milliseconds to wait=u32 1000) -> ()  [unwired: 1 out]
            }
            frame 1, Default {
              n232 = local read "Data Format"() -> (w453:T23)
              n233 = call "Save Data Functional Global.vi"("States"=Saving_Data_States."Save Data", "Data Format"=w453) -> ("error out"=w448:errorcluster)  [unwired: 6 in, 3 out]
              n234 = call "Save Data Functional Global.vi"("States"=Saving_Data_States."Get Queue Size", "error in (no error)"=w448) -> ("error out"=w447:errorcluster, "# elements in queue"=w449:i32)  [unwired: 6 in, 2 out]
              n235 = Equal To 0?(x=w449) -> (x = 0?=w450:bool)
            }
          }
        }
        n236 = while {
          tunnel: w431 -> [_]
          tunnel: w433 -> [w467]
          shift-right: [ATS_Async_Ctrl."Get" ("ATS_Async_Ctrl")] -> _
          shift-left: ATS_Async_Ctrl."StartCapture" ("ATS_Async_Ctrl") -> [w464]
          tunnel: w411 -> [w456]
          tunnel: w409 -> [w455]
          stop <- w454 stop-if-true
          n237 = call "ATS_AsyncDMA_Device.vi"("DeviceIn"=w467, "ATS_Async_Ctrl"=w464) -> ("Buffer"=w460:u16[], "Async_Status"=w462:T5)  [unwired: 9 in, 3 out]
          n238 = Unbundle By Name(w462) -> ("Valid"=w461:bool, "Completed"=w457:bool, "Start DMA"=w458:bool, "Timeout"=w466:bool, "Error"=w465:bool)
          n239 = local read "Reset DAQ"() -> (w459:bool)
          n240 = Compound Arithmetic op=OR(w457, invert w458, w466, w465, w459) -> (w454:bool)
          n241 = case shown="True" w461 {
            tunnel: w460 -> [_ w470]
            tunnel: w460 -> [_ w471]
            tunnel: w456 -> [_ w472]
            tunnel: w455 -> [_ w469]
            frame False {
              # "Do nothing"
            }
            frame True {
              w468 = 50 ("timeout in ms (-1)")
              n242 = Enqueue Element(queue=w469, element=w470, timeout in ms (-1)=w468) -> ()  [unwired: 1 in, 3 out]
              n243 = Enqueue Element(queue=w472, element=w471, timeout in ms (-1)=w468) -> ()  [unwired: 1 in, 3 out]
            }
          }
        }
        n244 = call "Save Data Functional Global.vi"("States"=Saving_Data_States."Close Files", "error in (no error)"=w421) -> ("error out"=w420:errorcluster)  [unwired: 6 in, 3 out]
        n245 = call "Save Data Functional Global.vi"("States"=Saving_Data_States."Do Nothing" ("Save State"), "error in (no error)"=w420) -> ("error out"=w418:errorcluster)  [unwired: 6 in, 3 out]
        n246 = Enqueue Element(queue=w425, element=OCT_Hardware_States."Stop", error in (no error)=w418) -> ()  [unwired: 1 in, 3 out]
      }
      frame "Set Resampling Array" {
        n247 = Wait (ms)(milliseconds to wait=u32 10) -> ()  [unwired: 1 out]
      }
      frame "Stop" {
        n248 = Release Queue(queue=w484, error in (no error)=w483) -> (error out=w482:errorcluster)  [unwired: 1 in, 2 out]
        n249 = call "OCT Processing 2ch functional global.vi"("State"=processing_states."Shutdown", "error in (no error)"=w482) -> ("error out"=w481:errorcluster)  [unwired: 5 in, 4 out]
        n250 = call "Save Data Functional Global.vi"("States"=Saving_Data_States."Shutdown", "error in (no error)"=w481) -> ("error out"=w478:errorcluster)  [unwired: 6 in, 3 out]
        n251 = call "galvo_functional_global.vi"("State"=galvo_states."Shutdown", "error in (no error)"=w478) -> ("error out"=w477:errorcluster)  [unwired: 8 in, 1 out]
        n252 = flat-sequence {
          tunnel: w477 -> [_]
          frame #0 {
            w488 = 0 ("DeviceIn")
            n253 = call "ATS_AsyncDMA_Device.vi"("DeviceIn"=w488, "ATS_Async_Ctrl"=ATS_Async_Ctrl."Stop") -> ("ReadSamples_Out"=w487:T37)  [unwired: 9 in, 4 out]
            n254 = call "ATS_AsyncDMA_Device.vi"("DeviceIn"=w488, "ATS_Async_Ctrl"=ATS_Async_Ctrl."Abort", "ReadSamples"=w487) -> ()  [unwired: 8 in, 5 out]
          }
          frame #1 {
            n255 = Stop(stop? (T)=TRUE) -> ()
          }
        }
      }
      frame "Set Clock" {
        w493 = T15 12 items=["20mV", "40mV", "50mV", "80mV", "100mV", "200mV", "400mV", "500mV", "800mV", "1 V", "1.25 V", "2 V", "4 V", "5 V", "8 V", "10 V", "16 V", "20 V", "40 V", "HiFi"] ("Input B.Range")
        w496 = u32 18 items=["1 kS/s", "2 kS/s", "5 kS/s", "10 kS/s", "20 kS/s", "50 kS/s", "100 kS/s", "200 kS/s", "500 kS/s", "1 MS/s", "2 MS/s", "5 MS/s", "10 MS/s", "20 MS/s", "50 MS/s", "100 MS/s", "125 MS/s", "160 MS/s", "180 MS/s"] ("ClckRate")
        n256 = local read "Clock Length"() -> (w495:u32)
        n257 = call "ATS_Device.vi"("BoardToVerify"=w491, "ATS_Check"=ATS_Check_Ctrl."Verify Board", "DevCtrl"=Device_Ctrl."Initialize", "DeviceIn"=0 ("Device")) -> ("error out"=w498:errorcluster, "DeviceOut"=w503:i32)  [unwired: 1 in, 5 out]
        n258 = Bundle By Name(cluster=w490, "Record.Length"=w495, "Clock.ClckSource"=ClockSource."Internal", "Clock.ClckRate"=w496, "Input B.Range"=w493, "Input A.Impedance"=Impedance."50 ohms") -> (w494:T7)
        n259 = call "ATS_Device.vi"("error in (no error)"=w498, "DevCtrl"=Device_Ctrl."Abort", "DeviceIn"=w503) -> ("DeviceOut"=w501:i32)  [unwired: 2 in, 6 out]
        n260 = call "ATS_MS_Set_Device.vi"("Set_Manually (F)"=FALSE, "Setup_In"=w494, "DeviceIn"=w501) -> ()  [unwired: 3 in, 6 out]
      }
    }
  }
  n261 = Destroy User Event(user event=w10) -> ()  [unwired: 1 in, 1 out]
